vi "dBhelper.vi"(6 "Bz":dbl[](array[numeric]), 8 "Bx":dbl[](array[numeric]), 9 "(3-r^2)/2":dbl[](array[numeric]), 10 "rsq":dbl[](array[numeric]), 11 "X":dbl[](array[numeric]) format="%#_13g") -> (1 "dBzdx":dbl[](array[numeric]), 2 "dBydx":dbl[](array[numeric]), 3 "dBxdx":dbl[](array[numeric]))   [LabVIEW 2017]
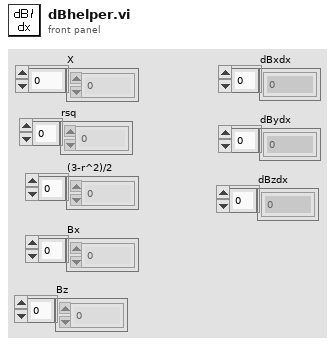
[diagram p1: front panel]
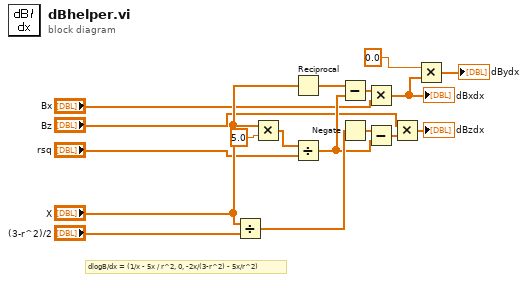
[diagram p0: block diagram]
diagram:
  # "dlogB/dx = (1/x - 5x / r^2, 0, -2x/(3-r^2) - 5x/r^2)"
  n1 = Divide(x="X", y="(3-r^2)/2") -> (x/y=w12:dbl[])
  n2 = Multiply(x="X", y=5.0) -> (x*y=w15:dbl[])
  n3 = Reciprocal(x="X") -> (1/x=w17:dbl[])
  n4 = Divide(x=w15, y="rsq") -> (x/y=w10:dbl[])
  n5 = Subtract(x=w17, y=w10) -> (x-y=w14:dbl[])
  n6 = Negate(x=w12) -> (-x=w11:dbl[])
  n7 = Multiply(x=w14, y="Bx") -> (x*y=w3:dbl[])
  "dBxdx" <- w3
  n8 = Subtract(x=w11, y=w10) -> (x-y=w9:dbl[])
  n9 = Multiply(x="Bz", y=w9) -> (x*y=→"dBzdx":dbl[])
  n10 = Multiply(x=0.0, y=w3) -> (x*y=→"dBydx":dbl[])
